vi "SVFA Cross Spectrum Subset (Mag-Phase).vi"(0 "scaled signal X [EUx]":waveform(dbl)={"t0"=timestamp(0 s since 1904-01-01), "dt"=1e-05, "Y"=[]}, 1 "scaled signal Y [EUy]":waveform(dbl)={"t0"=timestamp(0 s since 1904-01-01), "dt"=1e-05, "Y"=[]}, 2 "window":T11=1 items=["None"=0, "Hanning"=1, "Hamming"=2, "Blackman-Harris"=3, "Exact Blackman"=4, "Blackman"=5, "Flat Top"=6, "4 Term B-Harris "=7, "7 Term B-Harris"=8, "Low Sidelobe"=9, "Force - Exponential"=10, "Blackman Nuttall"=11, "Triangle"=30, "Bartlett-Hanning"=31, "Bohman"=32, "Parzen"=33, "Welch"=34, "Kaiser"=60, "Dolph-Chebyshev"=61, "Gaussian"=62], 3 "frequency range":T7={"start frequency"=1000.0, "stop frequency"=5000.0} {"stop frequency" min=0.0 format="%.2f"; "start frequency" min=0.0 format="%.2f"}, 4 "view":T9={"dB On (T)"=TRUE, "unwrap phase (F)"=FALSE, "convert to degree (T)"=TRUE}, 5 "error in (no error)":errorcluster, 7 "averaging parameters":T10={"averaging mode"=enum."No averaging", "weighting mode"=enum."Exponential", "number of averages"=10, "linear mode"=enum."One shot"}, 8 "force/exp settings":T8={"force window [%]"=50.0, "exp window [%]"=10.0} {"exp window [%]" min=0.0 max=100.0 format="%.2f"; "force window [%]" min=0.0 max=100.0 format="%.2f"}, 9 "restart averaging (F)":bool) -> (11 "averaging done":bool, 13 "averages completed":dbl, 14 "magnitude [dB EUx EUy]":cluster{"f0":dbl, "df":dbl, "magnitude":dbl[]}={"f0"=nan, "df"=inf, "magnitude"=[]} {"magnitude" format="%.2f"; "df" format="%.2f"; "f0" format="%.2f"}, 15 "magnitude unit label":string, 16 "phase [degrees]":cluster{"f0":dbl, "df":dbl, "phase":dbl[]}={"f0"=nan, "df"=inf, "phase"=[]} {"phase" format="%.2f"; "df" format="%.2f"; "f0" format="%.2f"}, 17 "phase unit label":string, 18 "spectrum info":T1={"channel name"="", "description"="", "x-axis units"=1, "spectral info"={"spectrum type"=enum."Power [Magnitude^2]", "linear/dB"=enum."linear", "window"=0, "window size"=0, "FFT size"=0}, "engineering units"=0, "custom label"="", "dB reference [EU]"=0.0, "peak units"=enum."rms", "weighting filter"=0, "spectral density?"=FALSE, "unit label"="", "spectrum skewed?"=FALSE, "complimentary spectrum units"=enum."none"} {"x-axis units" items=["Time (s)"=0, "Frequency-CB (Hz)"=1, "Frequency-CPB (Hz)"=1248, "Frequency-Arbitrary (Hz)"=2357, "Quefrency (s)"=2, "Revolutions (rev)"=3, "Order"=4, "Speed (RPM)"=11, "Speed (rad/s)"=21, "Index"=65535]; "weighting filter" items=["Linear", "A-weighting", "B-weighting", "C-weighting", "ITU-R 468-4", "Dolby", "CCITT", "C-message", "Wb", "Wc", "Wd", "We", "Wf", "Wh", "Wj", "Wk", "Wm", "AES17 20 kHz lowpass", "AES17 40 kHz lowpass", "AES17 20 kHz highpass", "AES17 40 kHz highpass"]; "dB reference [EU]" format="%.2f"; "engineering units" items=["custom..."=0, "V"=1, "A"=21, "C"=30, "pC"=31, "s"=32, "-"=29, "Pa"=2, "N"=20, "g"=3, "m/s^2"=4, "m/s"=5, "m"=6, "mm/s"=12, "mm"=13, "micron/s"=14, "micron"=15, "in/s^2"=7, "in/s"=8, "in"=9, "mil/s"=10, "mil"=11, "rad/s^2"=16, "rad/s"=17, "rad"=18, "deg/s^2"=26, "deg/s"=27, "deg"=28, "RPM"=22, "cycle/s^2"=23, "Hz"=24, "cycle"=25, "strain"=19]; "spectral info"."window" items=["None "=0, "Hanning"=1, "Hamming"=2, "Blackman-Harris"=3, "Exact Blackman"=4, "Blackman"=5, "Flat Top"=6, "4 Term B-Harris "=7, "7 Term B-Harris"=8, "Low Sidelobe"=9, "Force - Exponential"=10, "Gaussian"=62]}, 19 "error out":errorcluster)   [LabVIEW 2017]
doc: "Computes a subset of the cross power spectrum of <B>scaled signal X [EUx]</B> and <B>scaled signal Y [EUy]</B>. The subset is defined by <B>frequency range</B>. Results are returned as magnitude and phase."
uses:
  <vilib>/addons/_NISVFA/_Shared subVIs/Controls/svc_Window [Dual FFT].ctl
  <vilib>/addons/_NISVFA/_Shared subVIs/Controls/svc_Spectrum Info.ctl
  <vilib>/addons/_NISVFA/_Shared subVIs/Controls/svc_X-Axis Units.ctl
  <vilib>/addons/_NISVFA/_Shared subVIs/Controls/svc_Spectrum Type.ctl
  <vilib>/addons/_NISVFA/_Shared subVIs/Controls/svc_Engineering Units Text Ring.ctl
  <vilib>/addons/_NISVFA/_Shared subVIs/Controls/svc_Weighting Filter Text Ring.ctl
  <vilib>/addons/_NISVFA/_Shared subVIs/Controls/svc_Complimentary Spectrum Units.ctl
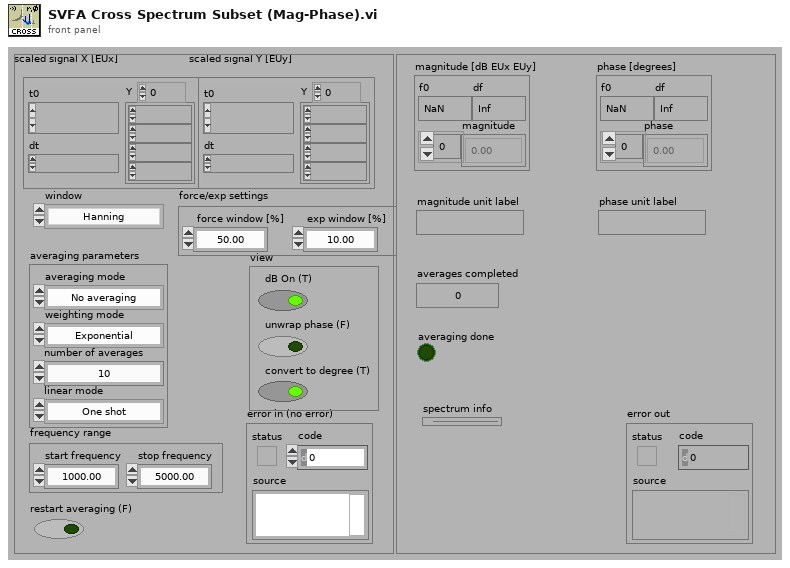
[diagram p1: front panel]
types:
  T1 = typedef "svc_Spectrum Info.ctl" = cluster{"channel name":string, "description":string, "x-axis units":T2, "spectral info":cluster{"spectrum type":T3, "linear/dB":enum16{"linear", "dB"}, "window":u16, "window size":i32, "FFT size":i32}, "engineering units":T4, "custom label":string, "dB reference [EU]":dbl, "peak units":enum16{"rms", "peak", "peak-peak"}, "weighting filter":T5, "spectral density?":bool, "unit label":string, "spectrum skewed?":bool, "complimentary spectrum units":T6}
  T2 = typedef "svc_X-Axis Units.ctl" = u16
  T3 = typedef "svc_Spectrum Type.ctl" = enum16{"FFT Spectrum [complex]", "Amplitude [Magnitude]", "Power [Magnitude^2]", "Cross Spectrum [complex]", "Frequency Response [Complex]"}
  T4 = typedef "svc_Engineering Units Text Ring.ctl" = u16
  T5 = typedef "svc_Weighting Filter Text Ring.ctl" = u16
  T6 = typedef "svc_Complimentary Spectrum Units.ctl" = enum16{"none", "radians", "degrees", "cycles", "imaginary"}
  T7 = cluster{"start frequency":dbl, "stop frequency":dbl}
  T8 = cluster{"force window [%]":dbl, "exp window [%]":dbl}
  T9 = cluster{"dB On (T)":bool, "unwrap phase (F)":bool, "convert to degree (T)":bool}
  T10 = cluster{"averaging mode":enum16{"No averaging", "Vector averaging", "RMS averaging", "Peak hold"}, "weighting mode":enum16{"Linear", "Exponential"}, "number of averages":u32, "linear mode":enum16{"One shot", "Auto restart"}}
  T11 = typedef "svc_Window [Dual FFT].ctl" = u32
  T12 = enum16{"Cross spectrum", "Frequency response", "Coherent output power"}
  T13 = enum16{"Restart processing", "Continue processing", "Skip processing"}
  T14 = cluster{"f0":dbl, "df":dbl, "complex spectrum":cdb[]}
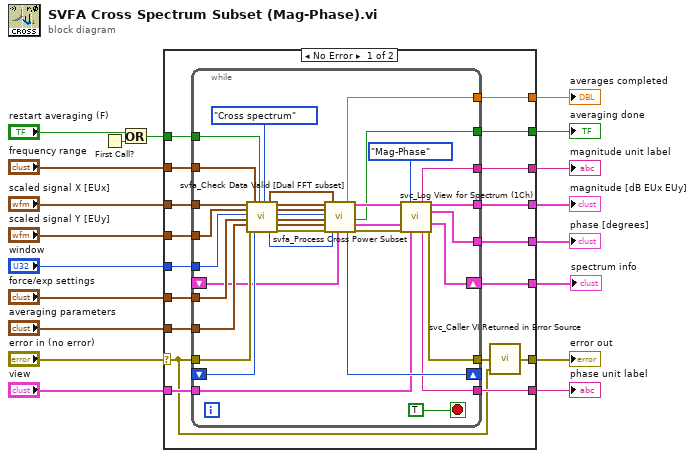
[diagram p0: block diagram]
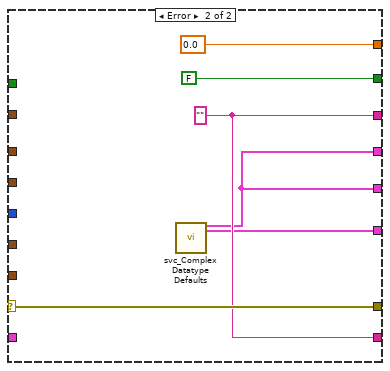
[diagram p2: hidden frame]
diagram:
  n1 = First Call?() -> (First Call?: T/F=w2:bool)
  n2 = Or(x="restart averaging (F)", y=w2) -> (x .or. y?=w1:bool)
  n3 = case shown="No Error" "error in (no error)" {
    selector: "error in (no error)" -> [w20 w77]
    tunnel: "window" -> [w35 _]
    tunnel: "averaging parameters" -> [w33 _]
    tunnel: "view" -> [w28 _]
    tunnel: [w21 w77] -> w16
    tunnel: [w24 w73] -> w15
    tunnel: [w25 w73] -> w14
    tunnel: "force/exp settings" -> [w34 _]
    tunnel: "scaled signal X [EUx]" -> [w37 _]
    tunnel: "scaled signal Y [EUy]" -> [w36 _]
    tunnel: w1 -> [w29 _]
    tunnel: [w26 w76] -> w8
    tunnel: [w23 w76] -> w7
    tunnel: [w30 0.0 ("averages completed")] -> w6
    tunnel: [w31 FALSE ("averaging done")] -> w5
    tunnel: "frequency range" -> [w32 _]
    tunnel: [w22 w72] -> w3
    frame No Error {
      n4 = while {
        tunnel: [w43] -> w23
        tunnel: [w44] -> w24
        tunnel: [w45] -> w25
        tunnel: [w46] -> w26
        tunnel: [w47] -> w27
        tunnel: w28 -> [w48]
        tunnel: w29 -> [w49]
        tunnel: [w57] -> w30
        tunnel: [w58] -> w31
        tunnel: w32 -> [w61]
        tunnel: w20 -> [w62]
        tunnel: w33 -> [w66]
        tunnel: w34 -> [w67]
        tunnel: w35 -> [w68]
        tunnel: w36 -> [w69]
        tunnel: w37 -> [w70]
        shift-left: _ -> [w65]
        shift-right: [w63] -> _
        shift-right: [w42] -> w22
        shift-left: _ -> [w39]
        stop <- TRUE stop-if-true
        n5 = call <vilib>:"svfa_Check Data Valid [Dual FFT subset].vi"("stimulus [X]"=w70, "response [Y]"=w69, "window"=w68, "force/exp settings"=w67, "averaging parameters"=w66, "error in (no error)"=w62, "frequency range"=w61, "processing control in"=w65, "restart averaging (F)"=w49, "measurement"=T12."Cross spectrum") -> ("dup frequency range"=w56:T7, "processing control out"=w64:T13, "dup stimulus [X]"=w55:waveform(dbl), "dup response [Y]"=w54:waveform(dbl), "window"=w53:u16, "dup force/exp settings"=w52:T8, "dup averaging parameters"=w51:T10, "error out"=w50:errorcluster)  [unwired: 1 in, 1 out]
        n6 = call <vilib>:"svfa_Process Cross Power Subset.vi"("Windowed signal [X]"=w55, "Windowed signal [Y]"=w54, "window"=w53, "force/exp settings"=w52, "averaging parameters"=w51, "error in (no error)"=w50, "Spectrum Settings"=w56, "processing control"=w64, "spectrum info in"=w39) -> ("averages completed"=w57:dbl, "processing control"=w63:T13, "complex spectrum"=w59:T14, "averaging done"=w58:bool, "spectrum info out"=w38:T1, "error out"=w40:errorcluster)  [unwired: 5 in]
        n7 = call <vilib>:"svc_Log View for Spectrum (1Ch).vi"("complex spectrum"=w59, "View"=enum16{"Mag-Phase", "Real-Imaginary"}."Mag-Phase", "spectrum info in"=w38, "error in (no error)"=w40, "view"=w48) -> ("unit label [mag or real]"=w46:string, "magnitude or real"=w45:cluster{"f0":dbl, "df":dbl, dbl[]}, "phase or imag"=w44:cluster{"f0":dbl, "df":dbl, dbl[]}, "spectrum info out"=w42:T1, "unit label [phase or imag]"=w43:string, "error out"=w47:errorcluster)  [unwired: 5 in]
      }
      n8 = call <vilib>:"svc_Caller VI Returned in Error Source.vi"("warning input to caller"=w20, "error in (no error)"=w27) -> ("error out"=w21:errorcluster)  [unwired: 3 in]
    }
    frame Error {
      w76 = "" ("Unit label [Mag - Real]")
      n9 = call <vilib>:"svc_Complex Datatype Defaults.vi"() -> ("empty spectrum"=w73:cluster{"f0":dbl, "df":dbl, "magnitude":dbl[]}, "dead spectrum info"=w72:T1)  [unwired: 11 in, 7 out]
    }
  }
  "error out" <- w16
  "phase [degrees]" <- w15
  "magnitude [dB EUx EUy]" <- w14
  "magnitude unit label" <- w8
  "phase unit label" <- w7
  "averages completed" <- w6
  "averaging done" <- w5
  "spectrum info" <- w3
